vi "Image affine transform.vi"(7 "method":i32(ring)=1 items=["nearest", "bilinear", "bicubic", "bicubic spline"], 8 "Affine array":dbl[](array[numeric]), 11 "Input image":i16[][](graph) caption="Detector A Low Mag") -> (3 "Output image":i16[][](graph) caption="Detector A Low Mag")   [LabVIEW 2018]
uses:
  <vilib>/gmath/interp.llb/Interpolate 2D (2d X,Y).vi
  <vilib>/gmath/NI_Gmath.lvlib
panel:
  out "Y array":i32[][](array[numeric])
  out "X array":i32[][](array[numeric])
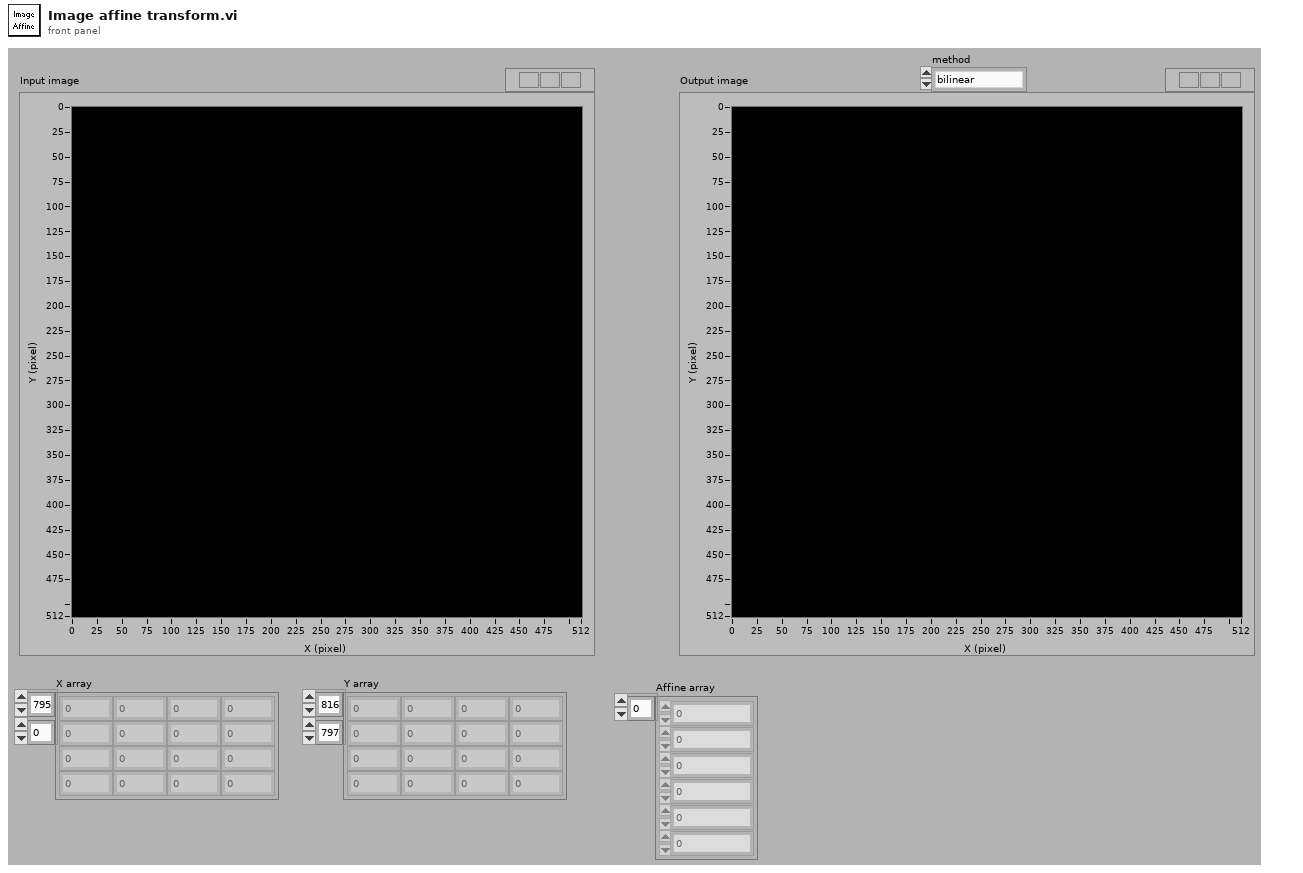
[diagram p1: front panel]
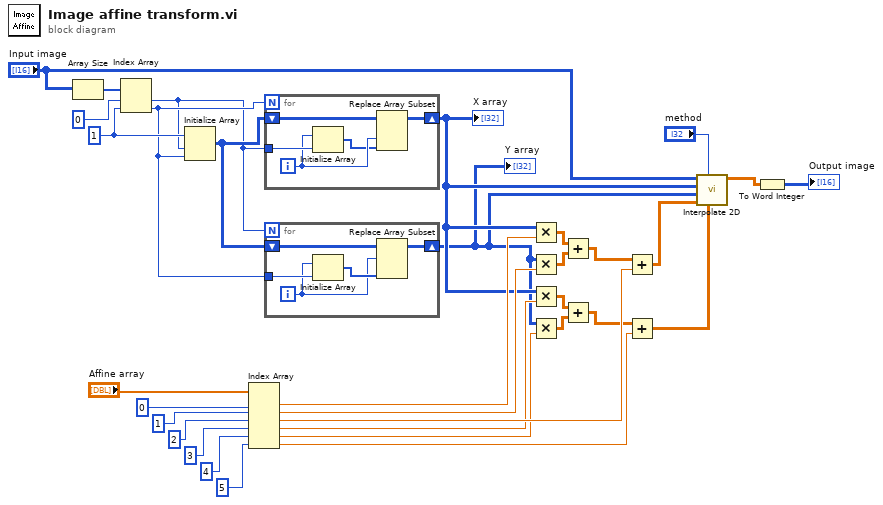
[diagram p0: block diagram]
diagram:
  w6 = 1 ("index")
  n1 = Array Size(array="Input image") -> (size(s)=w33:i32[])
  n2 = Index Array(array=w33, index #1=0 ("index"), index #2=w6) -> (element #1=w1:i32, element #2=w2:i32)
  n3 = Initialize Array(w6, w1, w2) -> (w4:i32[][])
  n4 = Index Array(array="Affine array", index #1=0 ("index"), index #2=1 ("index"), index #3=2 ("index"), index #4=3 ("index"), index #5=4 ("index"), index #6=5 ("index")) -> (element #1=w18:dbl, element #2=w16:dbl, element #3=w23:dbl, element #4=w12:dbl, element #5=w13:dbl, element #6=w24:dbl)
  n5 = for {
    N: w2 -> [_]
    shift-right: [w36] -> w5
    shift-left: w4 -> [w38]
    tunnel: w1 -> [w37]
    i -> [w35]
    n6 = Initialize Array(w35, w37) -> (w34:i32[])
    n7 = Replace Array Subset(array=w38, new element=w34, index (col)=w35) -> (w36:i32[][])  [unwired: 1 in]
  }
  "X array" <- w5
  n8 = for {
    N: w1 -> [_]
    shift-right: [w41] -> w3
    shift-left: w4 -> [w43]
    tunnel: w2 -> [w42]
    i -> [w39]
    n9 = Initialize Array(w39, w42) -> (w40:i32[])
    n10 = Replace Array Subset(array=w43, new element=w40, index (row)=w39) -> (w41:i32[][])  [unwired: 1 in]
  }
  "Y array" <- w3
  n11 = Multiply(x=w5, y=w18) -> (x*y=w17:dbl[][])
  n12 = Multiply(x=w3, y=w16) -> (x*y=w15:dbl[][])
  n13 = Multiply(x=w5, y=w12) -> (x*y=w10:dbl[][])
  n14 = Multiply(x=w3, y=w13) -> (x*y=w9:dbl[][])
  n15 = Add(x=w17, y=w15) -> (x+y=w14:dbl[][])
  n16 = Add(x=w10, y=w9) -> (x+y=w11:dbl[][])
  n17 = Add(x=w14, y=w23) -> (x+y=w8:dbl[][])
  n18 = Add(x=w11, y=w24) -> (x+y=w7:dbl[][])
  n19 = call-poly <vilib>:"Interpolate 2D.vi"("yi"=w7, "method"="method", "xi"=w8, "Y"=w3, "X"=w5, "Z"="Input image") -> ("zi"=w26:dbl[][])  [unwired: 2 in, 3 out]
  n20 = To Word Integer(number=w26) -> (16bit integer=→"Output image":i16[][])
